vi "Get Available Software.vi"   [LabVIEW 2017, in "nisyscfg.lvlib"]
doc: "Retrieves a list of software on the local system that is available for installation on a Real-Time target."
uses:
  <vilib>/nisyscfg/nisyscfg.lvlib
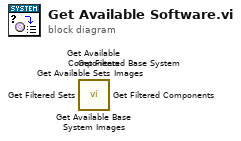
[diagram p0: block diagram]
diagram:
  n1 = call <vilib>:"Get Available Base System Images.vi"() -> ()  [unwired: 9 in, 3 out]
  n2 = call <vilib>:"Get Filtered Base System Images.vi"() -> ()  [unwired: 9 in, 3 out]
  n3 = call <vilib>:"Get Filtered Sets.vi"() -> ()  [unwired: 9 in, 3 out]
  n4 = call <vilib>:"Get Filtered Components.vi"() -> ()  [unwired: 9 in, 3 out]
  n5 = call <vilib>:"Get Available Sets.vi"() -> ()  [unwired: 9 in, 3 out]
  n6 = call <vilib>:"Get Available Components.vi"() -> ()  [unwired: 9 in, 3 out]
